vi "JSONRPC-InvokeJSON.vi"(8 "error in":errorcluster, 10 "variables":string, 11 "expid":string="\"%s\"") -> (0 "error out":errorcluster, 3 "response":string)   [LabVIEW 2014]
doc: "Parse a JSONRPC 2.0 string and invokes the corresponding method."
panel:
  in  "method":T1(ring)=enum."get"
  # "InvokeJSON"
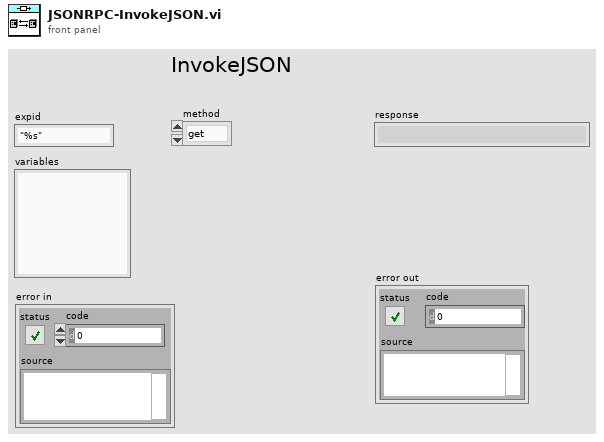
[diagram p1: front panel]
types:
  T1 = enum16{"open", "close", "start", "stop", "get", "set", "info", "UNDEFINED"}
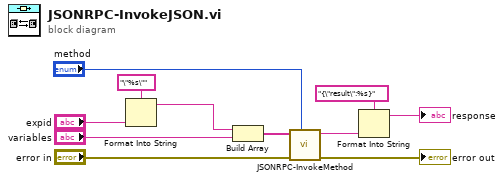
[diagram p0: block diagram]
diagram:
  n1 = Format Into String(format string="\"%s\"", "expid") -> (resulting string=w8:string)  [unwired: 2 in, 1 out]
  n2 = Build Array(w8, "variables") -> (w7:string[])
  n3 = call "JSONRPC-InvokeMethod.vi"("method"="method", "error in (no error)"="error in", "params"=w7) -> ("error out"=→"error out":errorcluster, "result"=w3:string)  [unwired: 7 in]
  n4 = Format Into String(format string="{\"result\":%s}", w3) -> (resulting string=→"response":string)  [unwired: 2 in, 1 out]
